vi "Append to Array - 1D Array String.vi"(8 "error in (no error)":errorcluster, 10 "1D String":string[](array[string]), 11 "JSON Tree in (JSON Array)":variant) -> (0 "error out":errorcluster, 3 "JSON Tree out (JSON Array)":variant)   [LabVIEW 2013, in "i3-json.lvlib"]
doc: "Appends a 1D String array to the given array"
uses:
  i3-json.lvlib
  JSON Types/JSON Type.ctl
  JSON Types/JSON Compatible Type.ctl
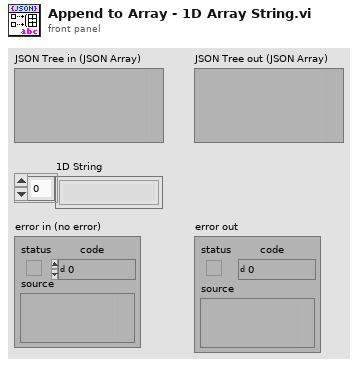
[diagram p1: front panel]
types:
  T1 = typedef "i3-json.lvlib/JSON Compatible Type.ctl" = enum16{"1D Double Array", "1D String Array", "1D Boolean Array", "Unknown"}
  T2 = typedef "i3-json.lvlib/JSON Type.ctl" = enum8{"JSON Compatible", "JSON Array", "JSON Object", "JSON Null", "Double", "String", "Boolean", "Unknown"}
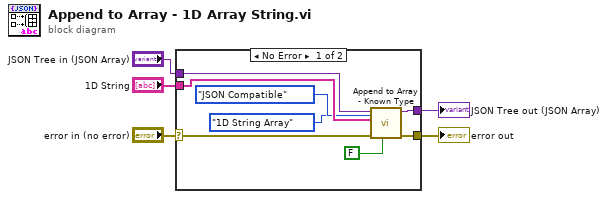
[diagram p0: block diagram]
diagram:
  n1 = case shown="No Error" "error in (no error)" {
    selector: "error in (no error)" -> [w11 w15]
    tunnel: [w12 w15] -> w4
    tunnel: [w13 w14] -> w3
    tunnel: "JSON Tree in (JSON Array)" -> [w10 w14]
    tunnel: "1D String" -> [w9 _]
    frame No Error {
      n2 = call "Append to Array - Known Type.vi"("JSON Compatible Type"=JSON_Compatible_Type."1D String Array", "Add Parameter as JSON Tree?"=FALSE, "JSON Type"=JSON_Type."JSON Compatible", "error in (no error)"=w11, "Value"=w9, "JSON Tree in (JSON Array)"=w10) -> ("error out"=w12:errorcluster, "JSON Tree out (JSON Array)"=w13:variant)  [unwired: 4 in]
    }
    frame Error {
    }
  }
  "error out" <- w4
  "JSON Tree out (JSON Array)" <- w3
